vi "InitiateAbortAll.vi"(8 "error in (no error)":errorcluster, 11 "TopLevel in":refnum<class "TopLevel.lvclass">) -> (0 "error out":errorcluster, 3 "TopLevel out":refnum<class "TopLevel.lvclass">)   [LabVIEW 2022 SP3, in "TopLevel.lvclass"]
uses:
  TopLevel.lvclass
  Motor Controller/Motor Controller.lvclass
  GIS Printer/GIS Printer.lvclass
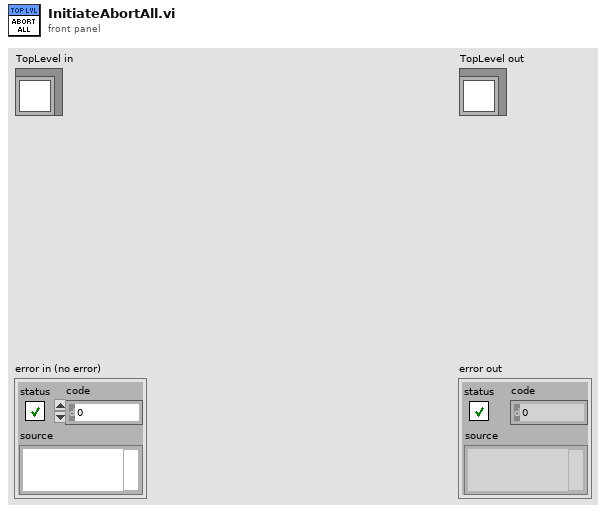
[diagram p1: front panel]
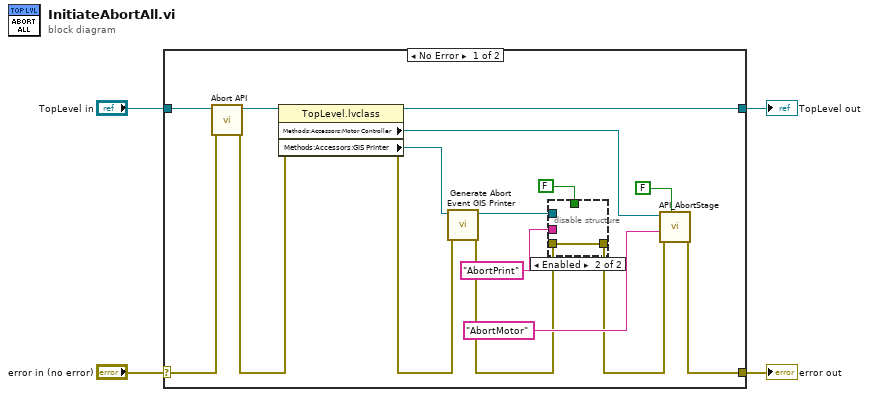
[diagram p0: block diagram]
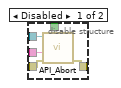
[diagram p2: hidden frame]
diagram:
  n1 = case shown="No Error" "error in (no error)" {
    selector: "error in (no error)" -> [w13 w28]
    tunnel: [w5 w28] -> w3
    tunnel: [w10 w27] -> w1
    tunnel: "TopLevel in" -> [w15 w27]
    frame No Error {
      n2 = call-dynamic "Abort API.vi"("error in (no error)"=w13, "TopLevel in"=w15) -> ("error out"=w9:errorcluster, "TopLevel out"=w14:refnum<class "TopLevel.lvclass">)  [unwired: 8 in]
      n3 = property class="TopLevel.lvclass"(reference=w14, error in=w9) -> (reference out=w10:refnum<class "TopLevel.lvclass">, error out=w8:errorcluster, "Methods:Accessors:Motor Controller"=w12:refnum<class "Motor Controller.lvclass">, "Methods:Accessors:GIS Printer"=w11:refnum<class "GIS Printer.lvclass">)
      n4 = call "Generate Abort Event GIS Printer.vi"("error in (no error)"=w8, "GIS Printer in"=w11) -> ("error out"=w7:errorcluster, "GIS Printer out"=w16:refnum<class "GIS Printer.lvclass">)  [unwired: 8 in]
      n5 = disable-structure shown="Enabled" {
        disable-tunnel: "AbortPrint" ("Task ID") -> [w25 _]
        disable-tunnel: FALSE ("Wait (F)") -> [w24 _]
        disable-tunnel: [w23 w26] -> w6
        disable-tunnel: w16 -> [w22 _]
        disable-tunnel: w7 -> [w21 w26]
        frame Disabled {
          n6 = call "API_Abort.vi"("Wait (F)"=w24, "error in (no error)"=w21, "Task ID"=w25, "GIS Printer in"=w22) -> ("error out"=w23:errorcluster)  [unwired: 5 in, 2 out]
        }
        frame Enabled {
        }
      }
      n7 = call "API_AbortStage.vi"("Wait (F)"=FALSE, "error in (no error)"=w6, "Task ID"="AbortMotor", "Motor Controller in"=w12) -> ("error out"=w5:errorcluster)  [unwired: 5 in, 2 out]
    }
    frame Error {
    }
  }
  "error out" <- w3
  "TopLevel out" <- w1
